vi "Main.vi"() -> ()   [LabVIEW 2015]
doc: "Use this template to build a simple state machine design pattern. Each state executes code and determines which state to transition to."
uses:
  controls/Data.ctl
  <vilib>/MakerHub/LINX/Private/Type Defs/LINX Ref.ctl
  <vilib>/MakerHub/LINX/Private/Type Defs/Platform.ctl
  <vilib>/MakerHub/LINX/Private/Type Defs/Interface.ctl
  <vilib>/MakerHub/LINX/Private/Device/Type Defs/LINX Device Config.ctl
  <vilib>/MakerHub/LINX/Private/Device/Type Defs/TCP Config.ctl
  <vilib>/MakerHub/LINX/Private/Device/Type Defs/Channels.ctl
  controls/State.ctl
  <vilib>/userdefined/High Color/IMAQdx.ctl
  <vilib>/vision/Avi.llb/IMAQ AVI2 Refnum.ctl
  <vilib>/vision/Avi.llb/IMAQ AVI2 Codec Path.ctl
  <vilib>/vision/driver/IMAQdx.llb/IMAQdx Camera Control Mode.ctl
  <vilib>/MakerHub/LINX/Private/Type Defs/User Platform.ctl
  <vilib>/MakerHub/LINX/Public/Peripherals/Digital/Digital Write 1 Chan.vi
  <vilib>/MakerHub/LINX/Public/Peripherals/Digital/Digital Write N Chans.vi
  <vilib>/MakerHub/LINX/Private/Local IO/LinxDigitalWrite.vi
  <vilib>/MakerHub/LINX/Public/Utilities/Check Channel.vi
  <vilib>/Instr/_visa.llb/VISA Configure Serial Port (Instr).vi
  <vilib>/MakerHub/LINX/Private/Utilties/Generate Error.vi
  <vilib>/MakerHub/LINX/LMH-LINX.lvlib
  <vilib>/vision/driver/NI_Vision_Acquisition_Software.lvlib
  <vilib>/measure/NI_MABase.lvlib
  <vilib>/MakerHub/LINX/Private/Device/Device.lvlib
panel:
  in  "Camera":T1="cam1"
  in  "Change Hopper Angle":bool
  in  "Hopper Angle":dbl=90.0
  in  "Left Hole Servo ID":u8=8
  in  "Right Hole Servo ID":u8=11
  in  "Table Tilt Servo ID":u8
  out "Current State":T2
  out "Data":T3={"LED"=FALSE, "Current State "="", "Current Angle"=0.0, "Angle Offset"=0.0, "Motor COM"="COM3", "Table Angle"=0.0, "LINX Ref"={"IO"=enum."Remote", "Interface"=enum."Serial", "LINX Device Config"={"Interface"=enum."Serial", "COM Port"="", "TCP Configuration"={"IP Address"="", "Port"=0}, "Device Family"=0, "Device ID"=0, "Device Name"="", "TCP Ref"=refnum, "Channels"={"DI"=[], "DO"=[], "AI"=[], "AO"=[], "PWM"=[], "QE"=[], "UART"=[], "I2C 2"=[], "SPI"=[], "CAN"=[], "Servo"=[], "AI Ref (V)"=0.0, "AI Resolution (Bits)"=0, "AO Ref (V)"=0.0, "AO Resolution (Bits)"=0}}}, "Mag-Filtered"={"X Axis"=0.0, "Y Axis"=0.0, "Z Axis"=0.0}, "G-Filtered"={"X Axis"=0.0, "Y Axis"=0.0, "Z Axis"=0.0}, "Desired Angle"=0.0, "Run Index"=0}
  in  "Start Automation":bool
  in  "Table Angle Array":dbl[](array[numeric])
  in  "Light LED":bool
  in  "Accelerometer Samples":i32=10
  in  "Save Frames":bool
  in  "Servo Incr":dbl=0.25
  in  "alpha":dbl=0.5 format="%#_13g"
  in  "Chip":enum16{"LSM6DS1", "LSM6DS3", "ADXL345"}(ring)=enum."ADXL345"
  in  "End video":bool=TRUE
  out "Start Video":bool=TRUE
  out "actual path":path
  out "Error Out":errorcluster
  out "Start Camera":bool=TRUE
  out "Camera In":T10(plugin-control)
  in  "Recalibrate":bool
  out "Current Table Angle":dbl
  in  "Motor COM":refnum<visa-resource-name>="COM10"
  in  "Arduino COM":refnum<visa-resource-name>="COM9"
  out "Device Name":string
  in  "Angle":dbl
  out "Current Servo Angle":dbl
  in  "Move To Angle":bool
  out "Exit":bool
  # "-90"
  # "-90"
  # "90"
  # "90"
  # "72 is FLAT!!!"
  # "Sim Controls"
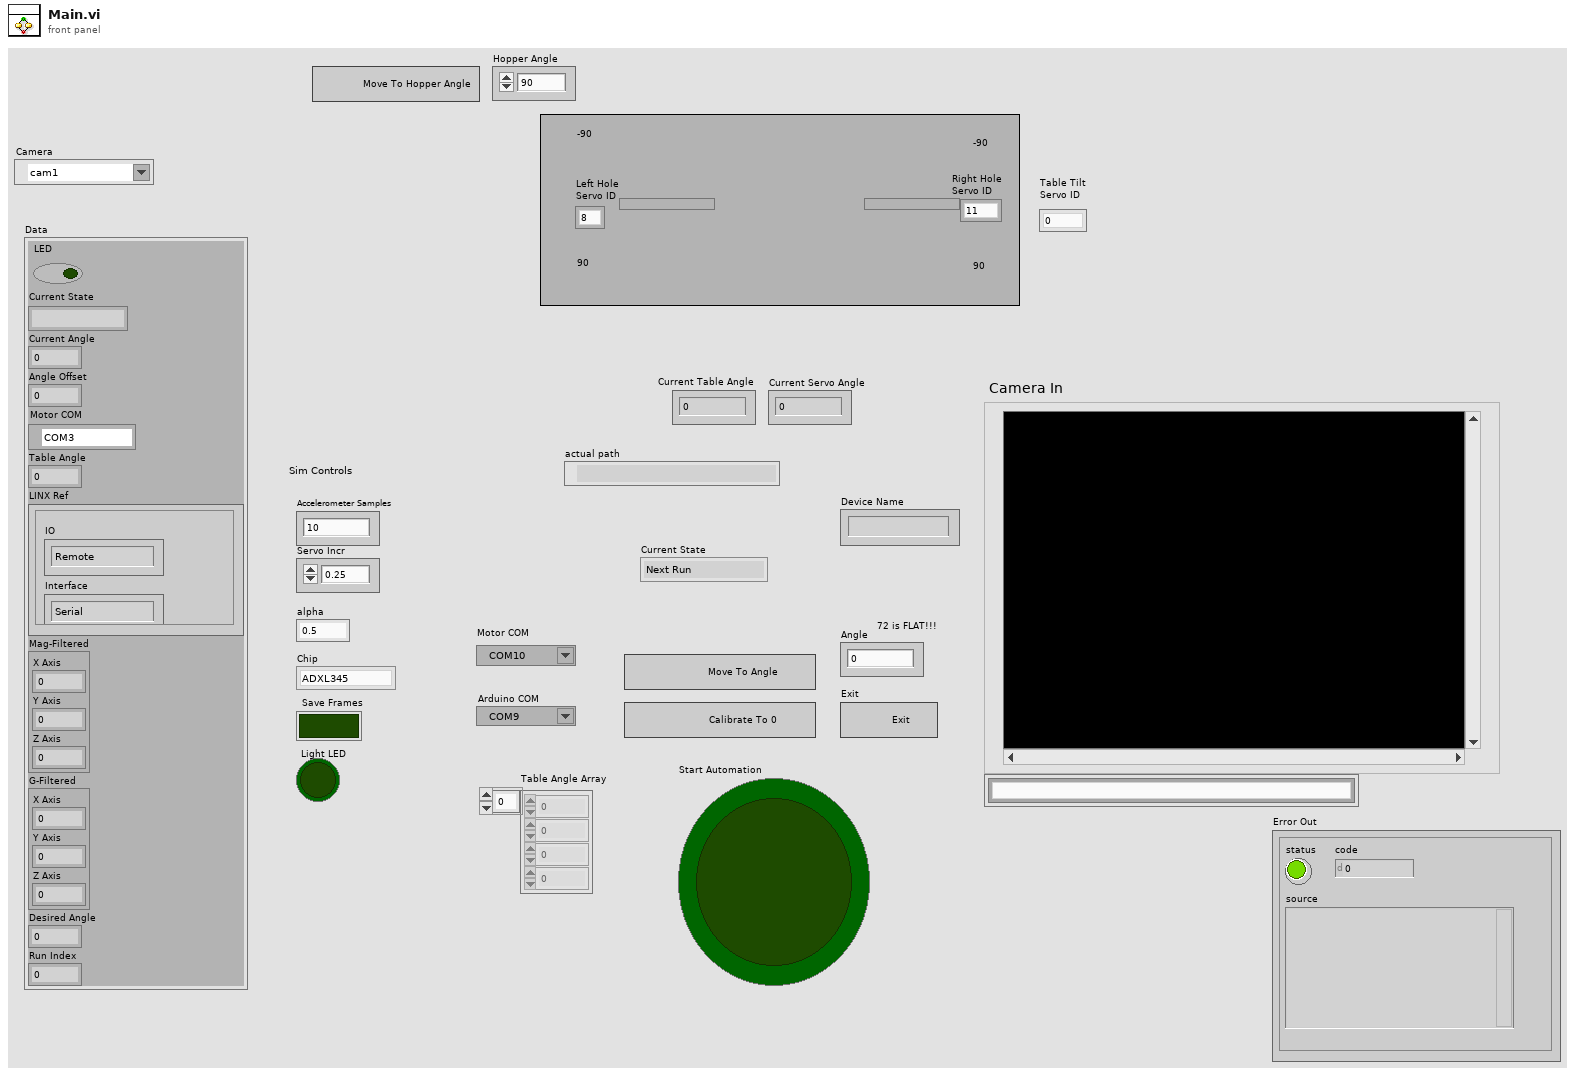
[diagram p1: front panel]
types:
  T1 = typedef "IMAQdx.ctl" = refnum<k21>
  T2 = typedef "State.ctl" = enum16{"Next Run", "Move To Angle (Auto)", "Initialize", "Initialize Camera", "Start Accelerometer", "Wait for Event", "User State 1", "User State 2", "Calibrate Angle", "Change Hole Angle", "Get Accelerometer Angle", "Move To Angle", "Play Tones", "Start Video", "End Video", "Move to 0", "Exit"}
  T3 = typedef "Data.ctl" = cluster{"LED":bool, "Current State ":string, "Current Angle":dbl, "Angle Offset":dbl, "Motor COM":refnum<visa-resource-name>, "Table Angle":dbl, "LINX Ref":T4, "Mag-Filtered":cluster{"X Axis":dbl, "Y Axis":dbl, "Z Axis":dbl}, "G-Filtered":cluster{"X Axis":dbl, "Y Axis":dbl, "Z Axis":dbl}, "Desired Angle":dbl, "Run Index":i32}
  T4 = typedef "LMH-LINX.lvlib/LINX Ref.ctl" = cluster{"IO":T5, "Interface":T6, "LINX Device Config":T7}
  T5 = typedef "LMH-LINX.lvlib/Platform.ctl" = enum16{"Remote", "Local"}
  T6 = typedef "LMH-LINX.lvlib/Interface.ctl" = enum16{"Serial", "TCP"}
  T7 = typedef "LMH-LINX.lvlib/Device.lvlib/LINX Device Config.ctl" = cluster{"Interface":T6, "COM Port":refnum<visa-resource-name>, "TCP Configuration":T8, "Device Family":u8, "Device ID":u8, "Device Name":string, "TCP Ref":refnum<k5>, "Channels":T9}
  T8 = typedef "LMH-LINX.lvlib/Device.lvlib/TCP Config.ctl" = cluster{"IP Address":string, "Port":u16}
  T9 = typedef "LMH-LINX.lvlib/Channels.ctl" = cluster{"DI":u8[], "DO":u8[], "AI":u8[], "AO":u8[], "PWM":u8[], "QE":u8[], "UART":u8[], "I2C 2":u8[], "SPI":u8[], "CAN":u8[], "Servo":u8[], "AI Ref (V)":dbl, "AI Resolution (Bits)":u8, "AO Ref (V)":dbl, "AO Resolution (Bits)":u8}
  T10 = typedef "IMAQ Image.ctl" = refnum<image>
  T11 = cluster{"X Axis":dbl, "Y Axis":dbl, "Z Axis":dbl}
  T12 = typedef "LMH-LINX.lvlib/User Platform.ctl" = enum16{"Default", "Remote", "Local"}
  T13 = typedef "IMAQ AVI2 Refnum.ctl" = refnum<k20>
  T14 = typedef "NI_Vision_Acquisition_Software.lvlib/IMAQdx Camera Control Mode.ctl" = enum32{"Controller", "Listener"}
  T15 = typedef "IMAQ AVI2 Codec Path.ctl" = u32
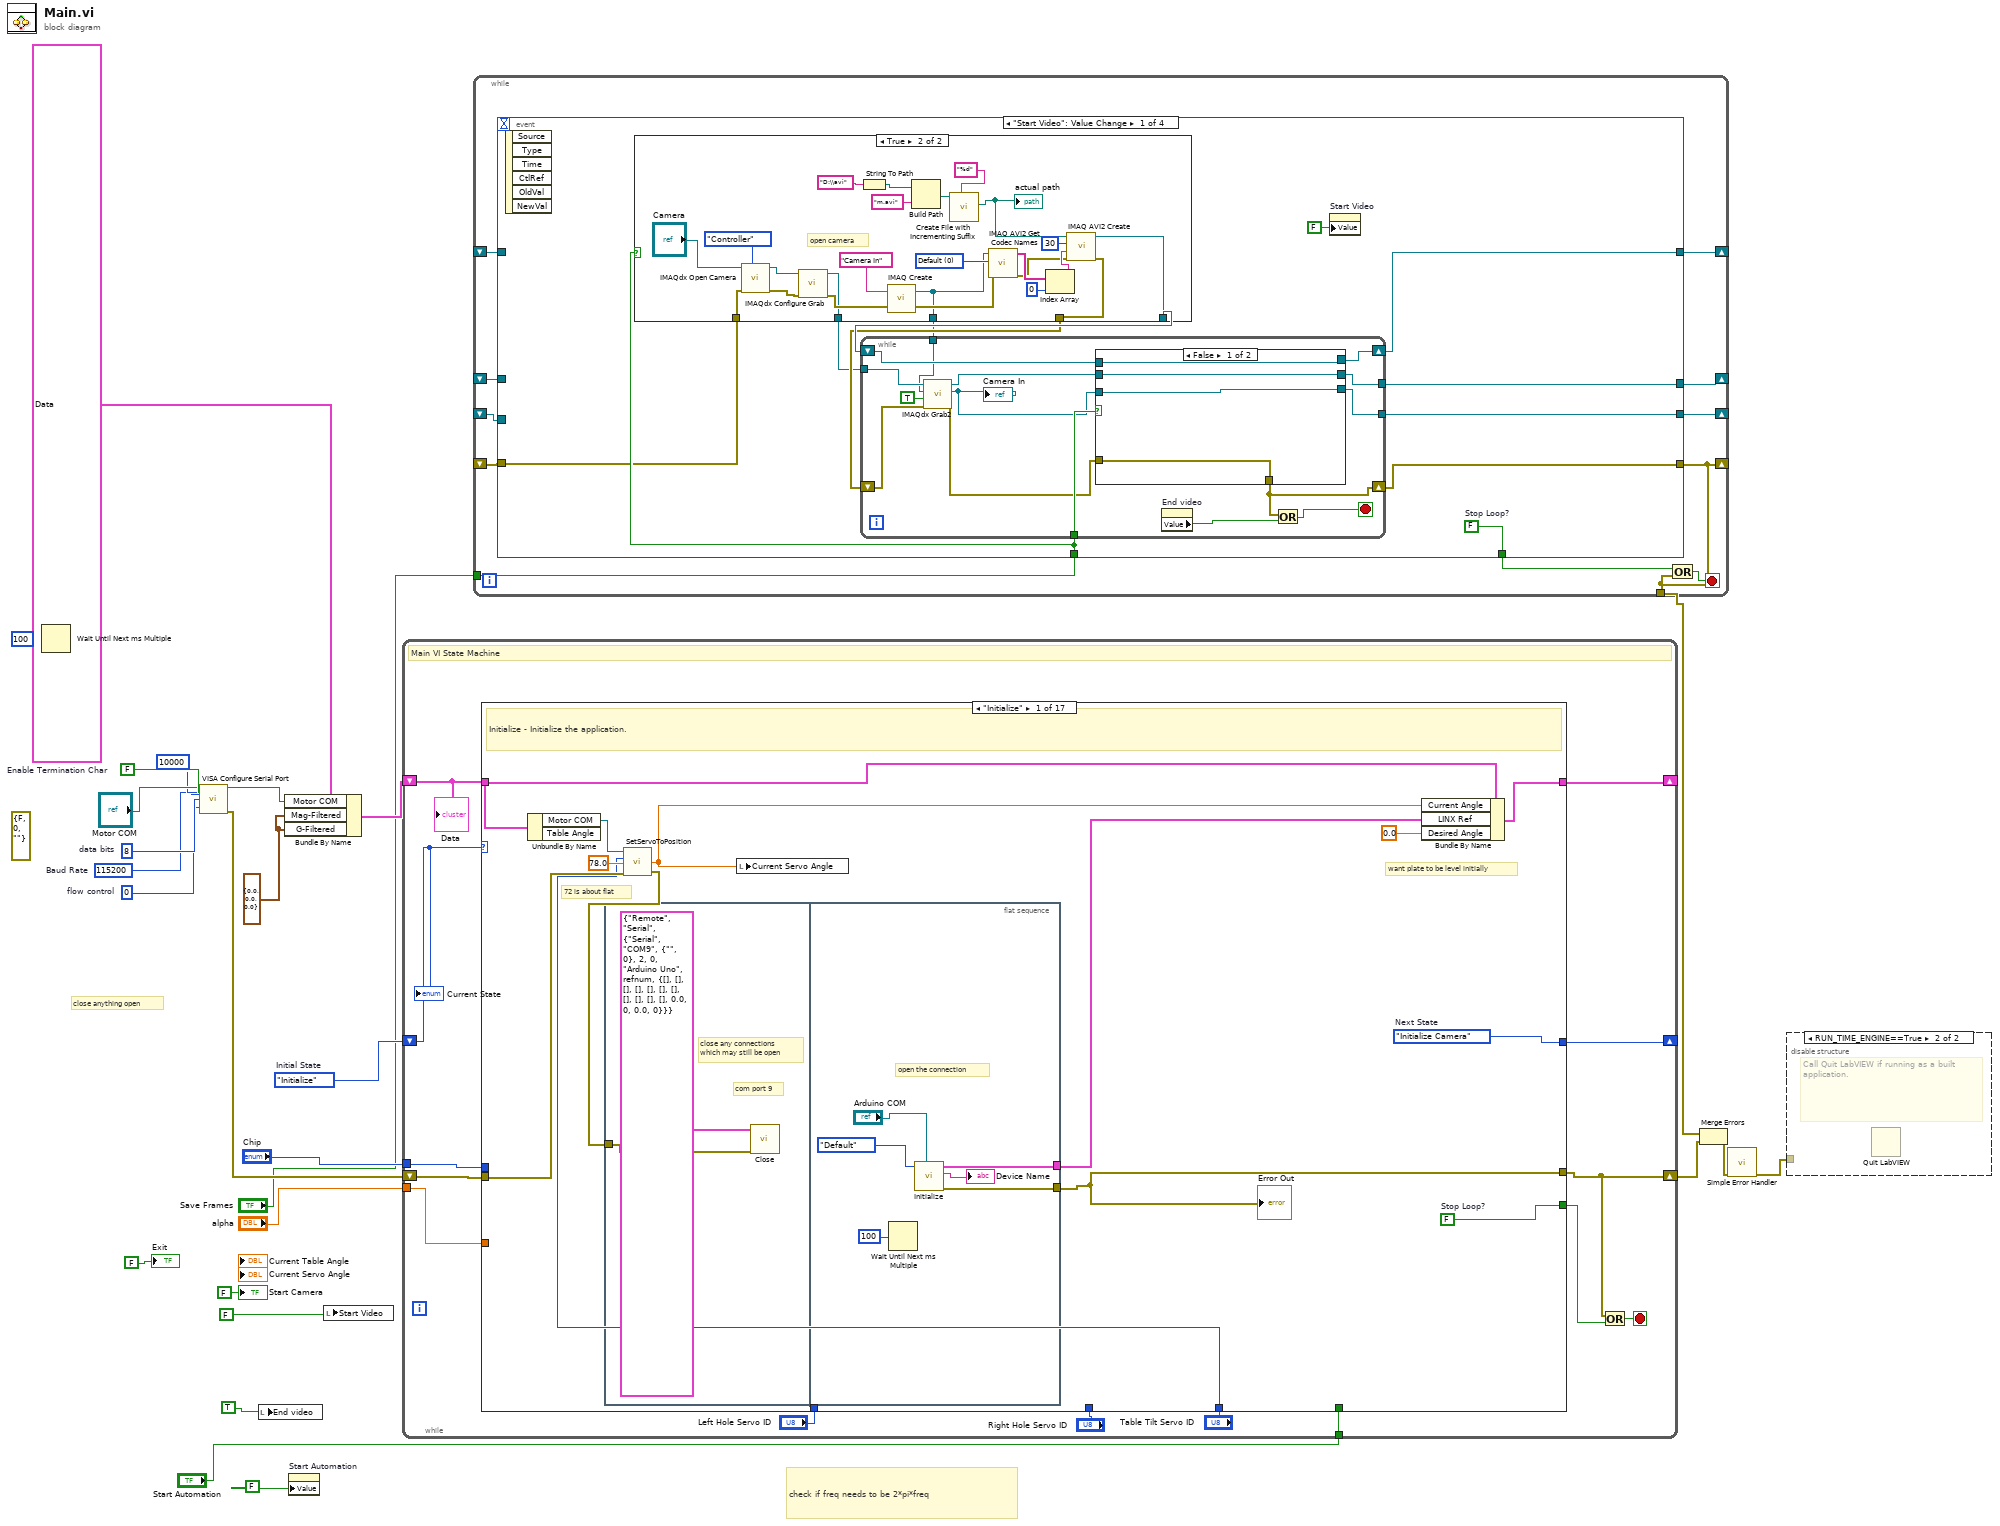
[diagram p0: block diagram]
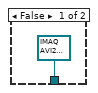
[diagram p2: hidden frame]
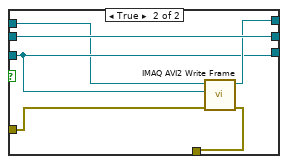
[diagram p3: hidden frame]
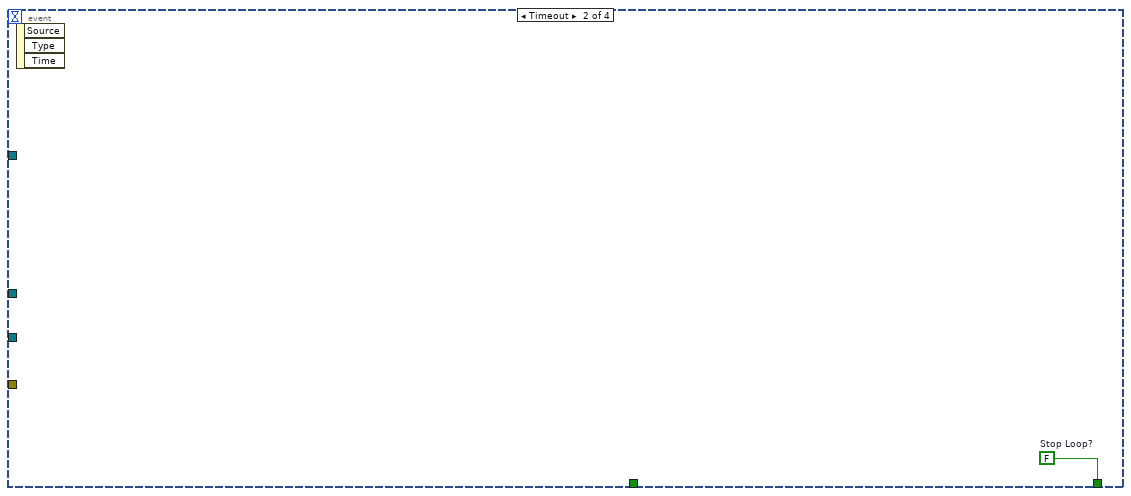
[diagram p4: hidden frame]
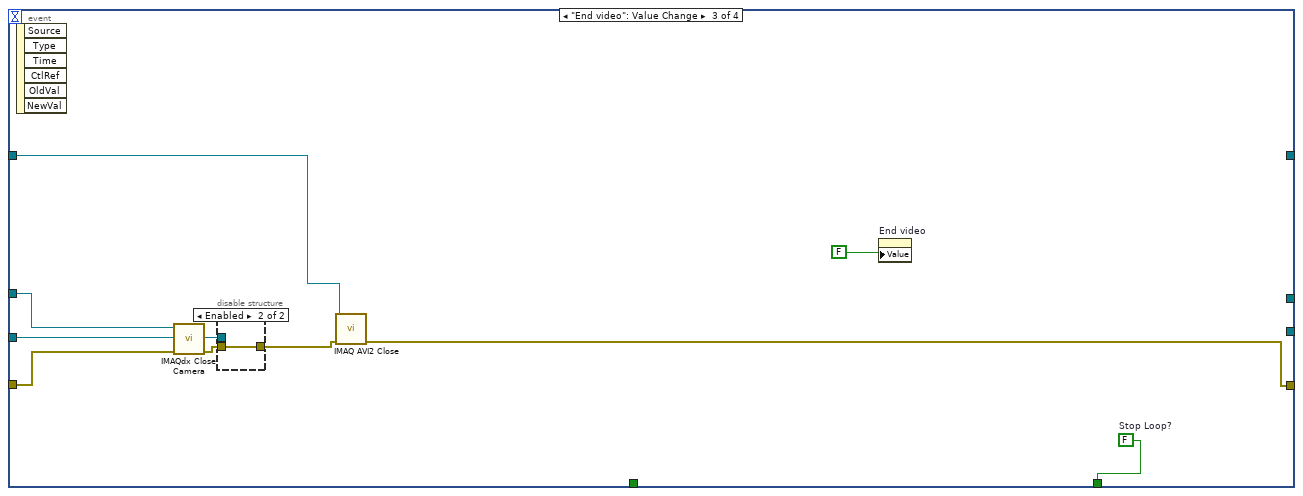
[diagram p5: hidden frame]
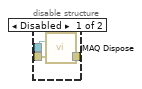
[diagram p6: hidden frame]
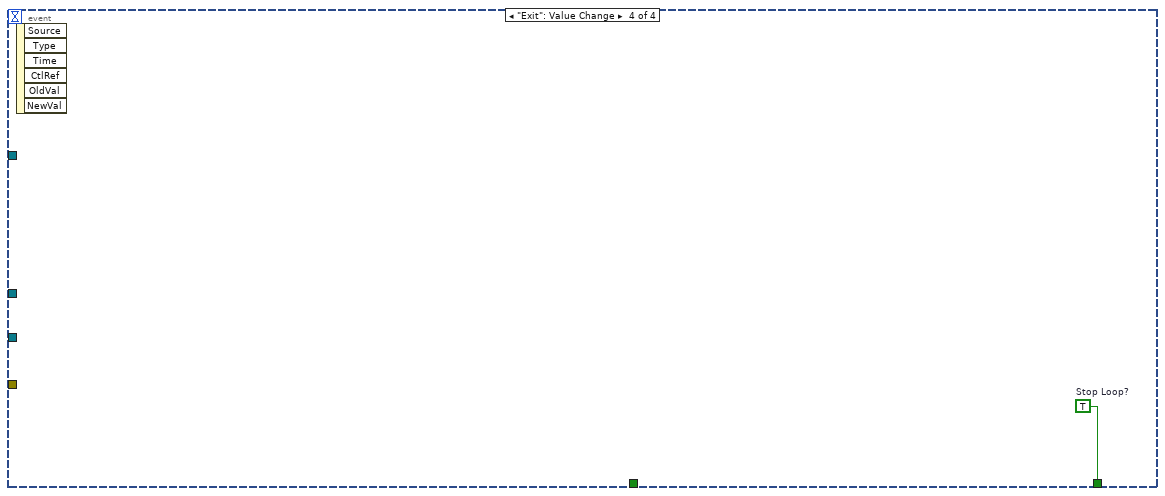
[diagram p7: hidden frame]
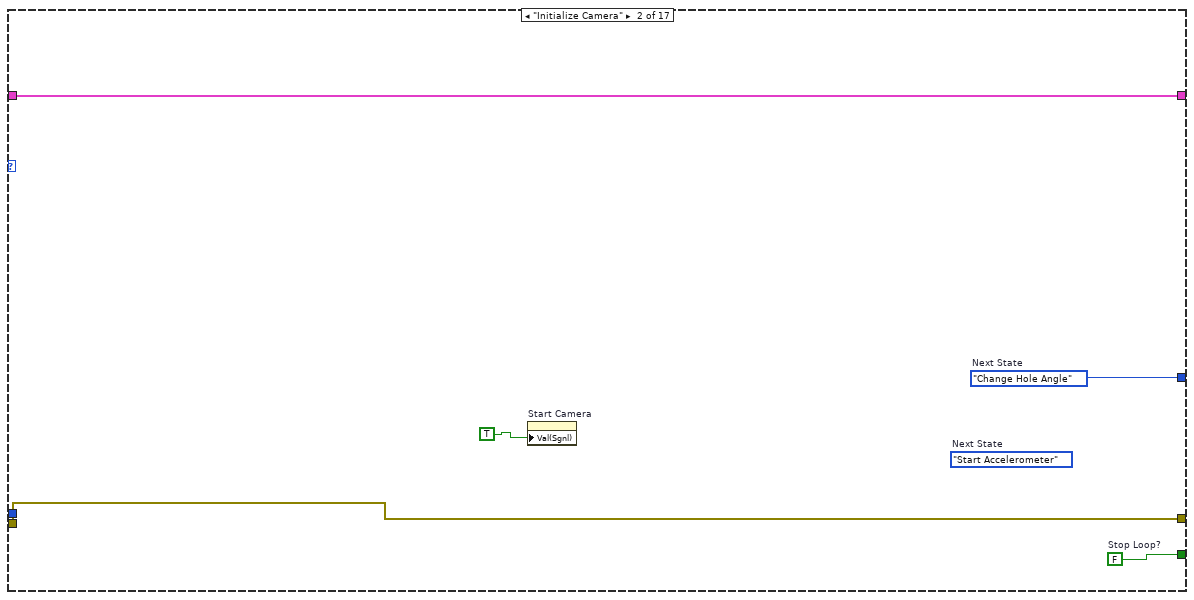
[diagram p9: hidden frame]
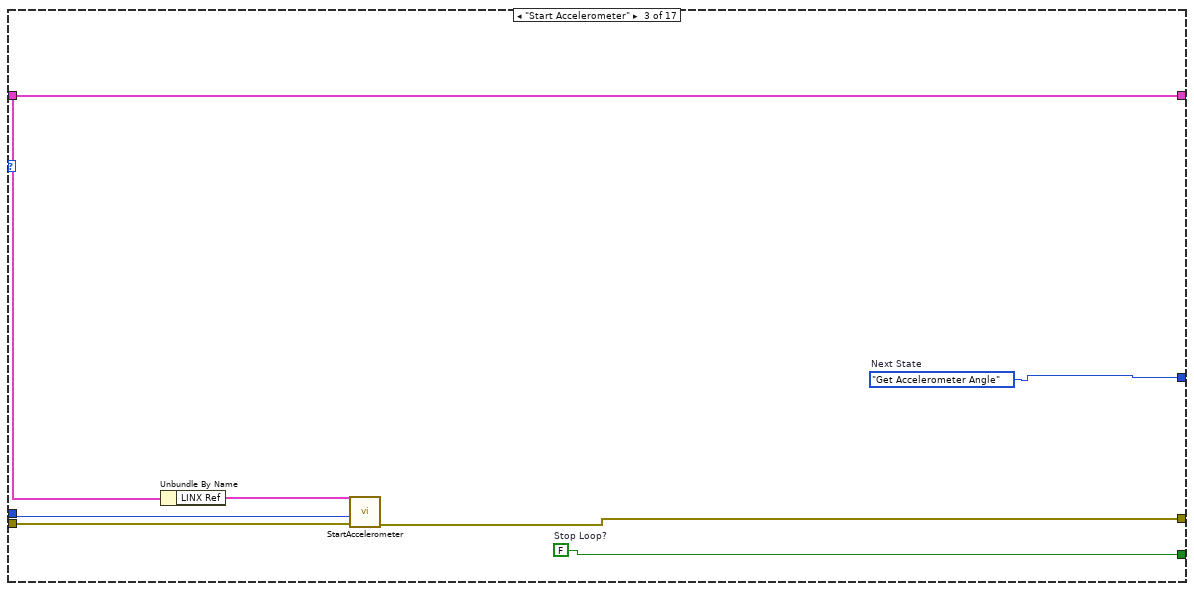
[diagram p10: hidden frame]
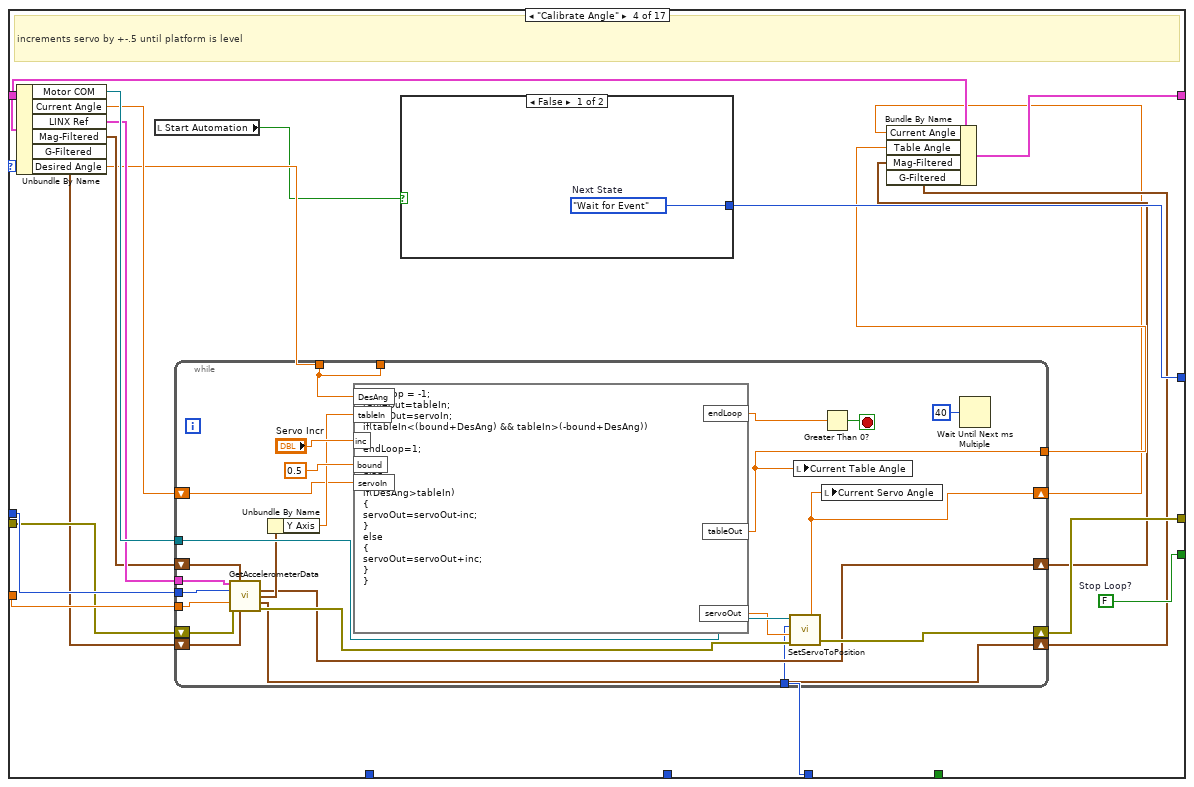
[diagram p11: hidden frame]
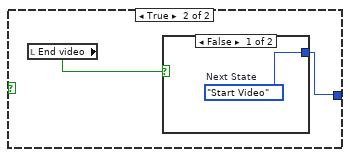
[diagram p12: hidden frame]
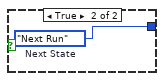
[diagram p13: hidden frame]
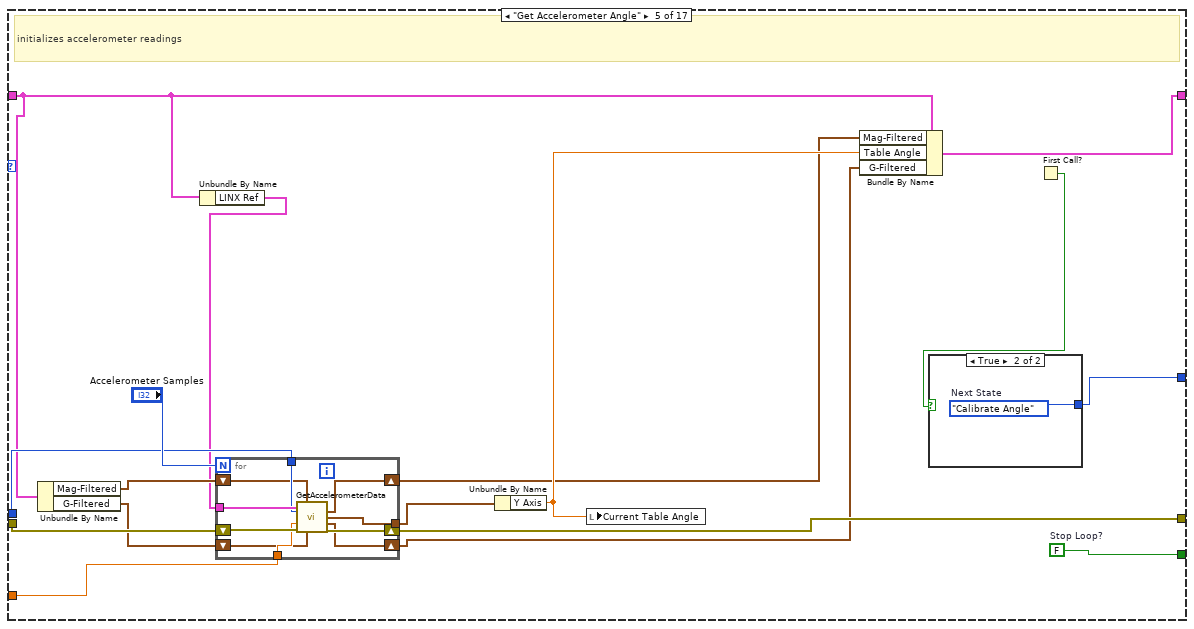
[diagram p14: hidden frame]
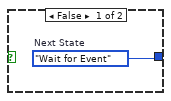
[diagram p15: hidden frame]
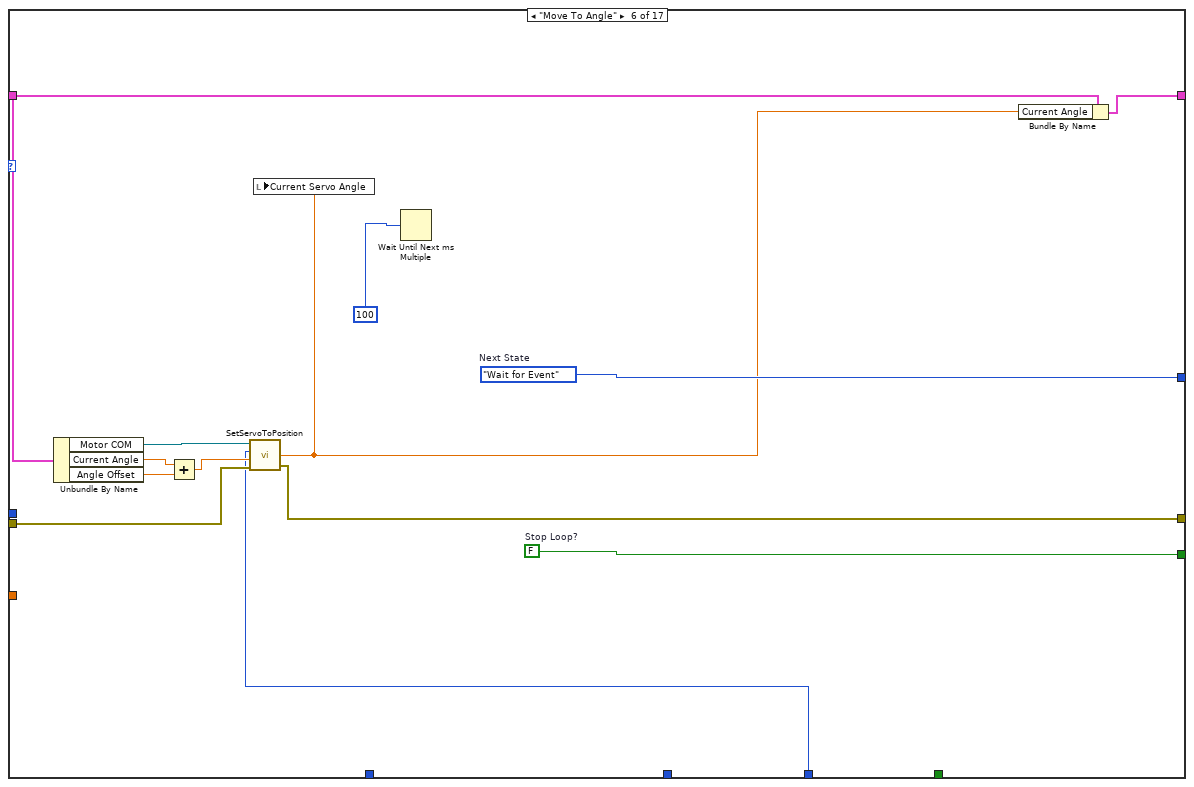
[diagram p16: hidden frame]
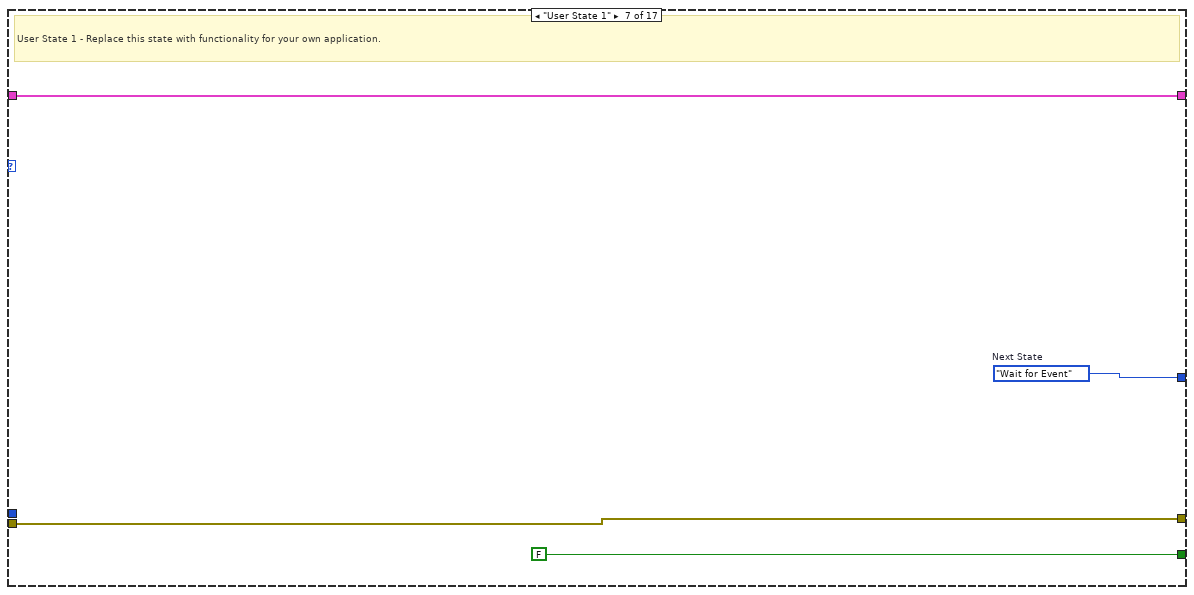
[diagram p17: hidden frame]
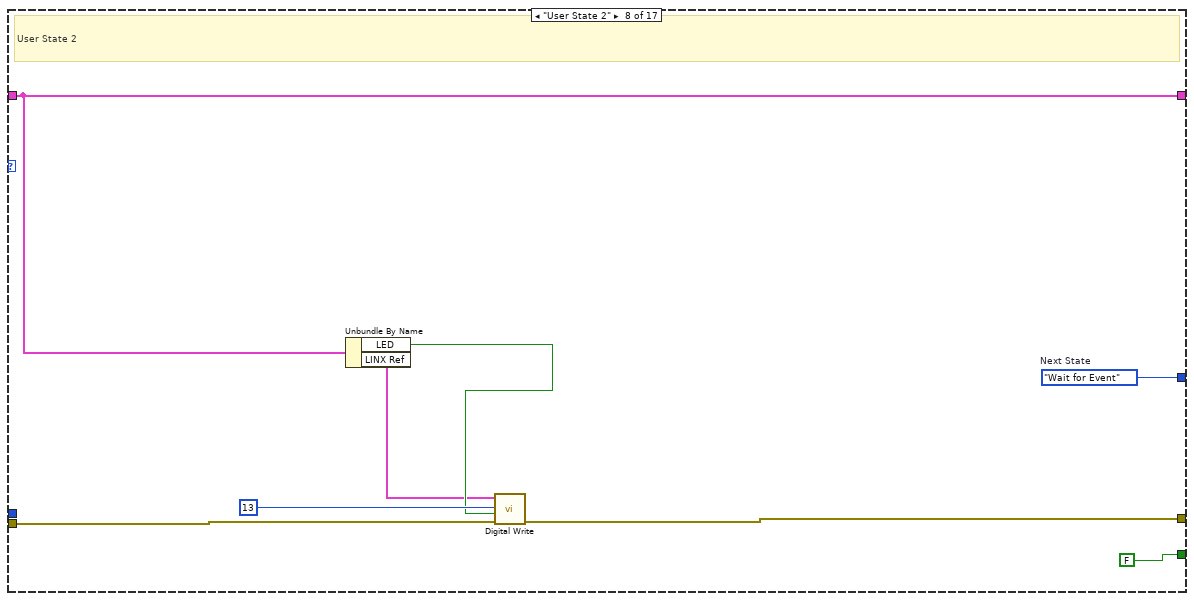
[diagram p18: hidden frame]
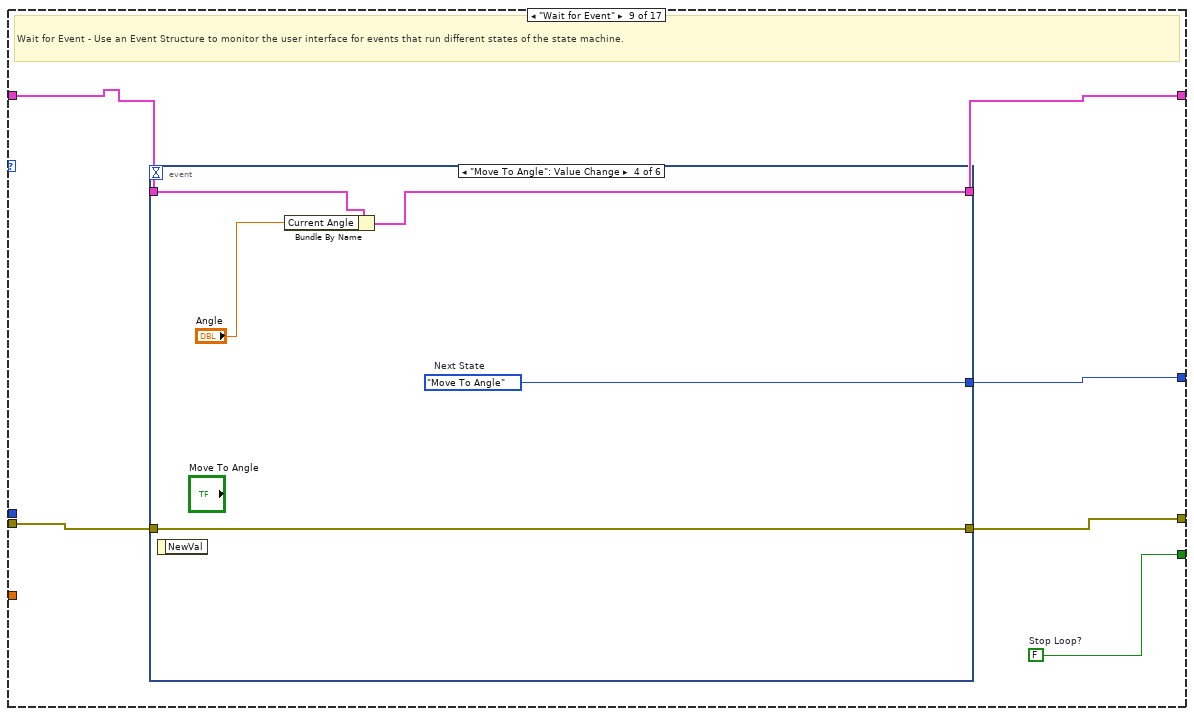
[diagram p19: hidden frame]
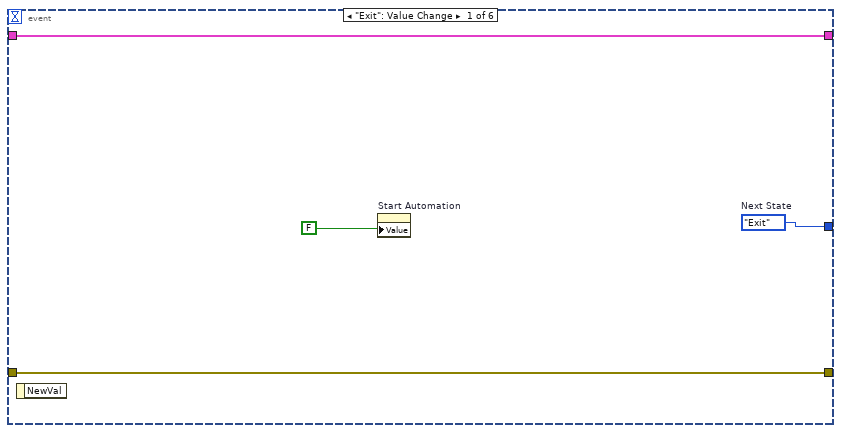
[diagram p20: hidden frame]
diagram:
  w14 = T11 {"X Axis"=0.0, "Y Axis"=0.0, "Z Axis"=0.0} ("Mag-Filtered")
  (unwired) errorcluster {"status"=FALSE, "code"=0, "source"=""} ("error out")
  w8 = u32 115200  # Baud Rate
  w22 = u16 0  # flow control
  w23 = u16 8  # data bits
  w24 = FALSE  # Enable Termination Char
  w20 = State."Initialize"  # Initial State
  # "check if freq needs to be 2*pi*freq"
  # "close anything open"
  n1 = Wait Until Next ms Multiple(millisecond multiple=u32 100) -> ()  [unwired: 1 out]
  n2 = call-poly "VISA Configure Serial Port"("VISA resource name"="Motor COM", "timeout (10sec)"=u32 10000, "Enable Termination\nChar (T)"=w24, "baud rate (9600)"=w8, "data bits (8)"=w23, "flow control (0:none)"=w22) -> ("VISA resource name out"=w7:refnum<visa-resource-name>, "error out"=w21:errorcluster)  [unwired: 8 in]
  n3 = local write "End video"(TRUE ("End video")) -> ()
  n4 = Bundle By Name(cluster=T3 {"LED"=FALSE, "Current State "="", "Current Angle"=0.0, "Angle Offset"=0.0, "Motor COM"="COM3", "Table Angle"=0.0, "LINX Ref"={"IO"=enum."Remote", "Interface"=enum."Serial", "LINX Device Config"={"Interface"=enum."Serial", "COM Port"="", "TCP Configuration"={"IP Address"="", "Port"=0}, "Device Family"=0, "Device ID"=0, "Device Name"="", "TCP Ref"=refnum, "Channels"={"DI"=[], "DO"=[], "AI"=[], "AO"=[], "PWM"=[], "QE"=[], "UART"=[], "I2C 2"=[], "SPI"=[], "CAN"=[], "Servo"=[], "AI Ref (V)"=0.0, "AI Resolution (Bits)"=0, "AO Ref (V)"=0.0, "AO Resolution (Bits)"=0}}}, "Mag-Filtered"={"X Axis"=0.0, "Y Axis"=0.0, "Z Axis"=0.0}, "G-Filtered"={"X Axis"=0.0, "Y Axis"=0.0, "Z Axis"=0.0}, "Desired Angle"=0.0, "Run Index"=0} ("Data"), "Motor COM"=w7, "Mag-Filtered"=w14, "G-Filtered"=w14) -> (w19:T3)
  n5 = property on="Start Automation" class="Bool (strict)"("Value"=FALSE ("End video")) -> ()  [unwired: 2 in, 2 out]
  n6 = local write "Start Video"(FALSE ("Start Video")) -> ()
  n7 = while {
    shift-right: [w40] -> _
    shift-left: w20 -> [w31]
    shift-right: [w39] -> _
    shift-left: w19 -> [w32]
    shift-right: [w35] -> w13
    shift-left: w21 -> [w38]
    tunnel: "Chip" -> [w34]
    tunnel: "alpha" -> [w33]
    tunnel: "Start Automation" -> [w27]
    stop <- w36 stop-if-true
    # "Main VI State Machine"
    n8 = case shown="\"Initialize\"" w31 {
      tunnel: [w53 w65 w67 w91 w138 w163 w168 w176 w182 w211 w224 State."End Video" ("Next State") w249 w264 w291 State."Next Run" ("(Value Not Used)") w308] -> w40
      tunnel: [w52 w66 w73 w93 w139 w164 FALSE ("Stop Loop?") FALSE ("Stop Loop?") w181 w222 w223 w235 w248 w265 w290 _ _] -> w37
      tunnel: w32 -> [w48 w64 w71 w87 w124 w158 w165 w169 w177 w213 w226 w237 w251 w259 w286 w293 w312]
      tunnel: [w49 w64 w71 w92 w130 w162 w165 w169 w180 w217 w226 w237 w251 w255 w286 w292 w312] -> w39
      tunnel: w38 -> [w46 w63 w69 w88 w136 w160 w166 w174 w179 w216 w225 w231 w250 w266 w288 w297 w318]
      tunnel: [w41 w63 w68 w85 w135 w159 w166 w173 w178 w215 w225 w230 w250 w266 w289 w297 w310] -> w35
      tunnel: w34 -> [_ _ w72 w90 w134 _ _ _ _ _ _ _ _ _ _ _ _]
      tunnel: w33 -> [_ _ _ w89 w133 _ _ _ _ _ _ _ _ _ _ _ _]
      tunnel: "Table Tilt Servo ID" -> [w42 _ _ w74 _ w152 _ _ _ w210 _ _ _ _ _ _ _]
      tunnel: "Right Hole Servo ID" -> [_ _ _ _ _ _ _ _ _ _ _ _ _ _ _ _ w319]
      tunnel: "Left Hole Servo ID" -> [_ _ _ _ _ _ _ _ _ _ _ _ _ _ _ _ w315]
      tunnel: w27 -> [_ _ _ _ _ _ _ _ _ _ _ w229 _ _ _ _ _]
      frame "Initialize" {
        w52 = FALSE  # Stop Loop?
        w53 = State."Initialize Camera"  # Next State
        # "want plate to be level initially"
        # "72 is about flat"
        # "Initialize - Initialize the application."
        n9 = Unbundle By Name(w48) -> ("Motor COM"=w50:refnum<visa-resource-name>)  [unwired: 1 out]
        n10 = flat-sequence {
          tunnel: w45 -> [w54]
          tunnel: [w58] -> w41
          tunnel: [w57] -> w44
          frame #0 {
            # "com port 9"
            # "close any connections\nwhich may still be open"
            n11 = call <vilib>:"Close.vi"("Error In"=w54, "LINX Resource"=T4 {"IO"=enum."Remote", "Interface"=enum."Serial", "LINX Device Config"={"Interface"=enum."Serial", "COM Port"="COM9", "TCP Configuration"={"IP Address"="", "Port"=0}, "Device Family"=2, "Device ID"=0, "Device Name"="Arduino Uno", "TCP Ref"=refnum, "Channels"={"DI"=[], "DO"=[], "AI"=[], "AO"=[], "PWM"=[], "QE"=[], "UART"=[], "I2C 2"=[], "SPI"=[], "CAN"=[], "Servo"=[], "AI Ref (V)"=0.0, "AI Resolution (Bits)"=0, "AO Ref (V)"=0.0, "AO Resolution (Bits)"=0}}} ("LINX Ref")) -> ()  [unwired: 9 in, 1 out]
          }
          frame #1 {
            # "open the connection"
            n12 = Wait Until Next ms Multiple(millisecond multiple=u32 100) -> ()  [unwired: 1 out]
            n13 = call <vilib>:"Initialize.vi"("Serial Port"="Arduino COM", "IO"=User_Platform."Default" ("Platform")) -> ("Error Out"=w58:errorcluster, "Device Name"=→"Device Name":string, "LINX Resource"=w57:T4)  [unwired: 7 in]
          }
        }
        n14 = call "SetServoToPosition.vi"("error in (no error)"=w46, "RF LF"=78.0, "servo channel"=w42, "VISA resource name"=w50) -> ("error out"=w45:errorcluster, "RF LF 2"=w47:dbl)  [unwired: 1 out]
        n15 = local write "Current Servo Angle"(w47) -> ()
        n16 = Bundle By Name(cluster=w48, "Current Angle"=w47, "LINX Ref"=w44, "Desired Angle"=0.0) -> (w49:T3)
        "Error Out" <- w41
      }
      frame "Initialize Camera" {
        (unwired) State."Start Accelerometer"  # Next State
        w65 = State."Change Hole Angle"  # Next State
        w66 = FALSE  # Stop Loop?
        n17 = property on="Start Camera" class="Bool (strict)"("Val(Sgnl)"=TRUE) -> ()  [unwired: 2 in, 2 out]
      }
      frame "Start Accelerometer" {
        w67 = State."Get Accelerometer Angle"  # Next State
        w73 = FALSE  # Stop Loop?
        n18 = Unbundle By Name(w71) -> ("LINX Ref"=w70:T4)
        n19 = call "StartAccelerometer.vi"("Error In"=w69, "Chip"=w72, "LINX Resource"=w70) -> ("Error Out"=w68:errorcluster)  [unwired: 3 in, 1 out]
      }
      frame "Calibrate Angle" {
        w93 = FALSE  # Stop Loop?
        # "increments servo by +-.5 until platform is level"
        n20 = Unbundle By Name(w87) -> ("Motor COM"=w86:refnum<visa-resource-name>, "Current Angle"=w84:dbl, "LINX Ref"=w83:T4, "Mag-Filtered"=w81:T11, "G-Filtered"=w79:T11, "Desired Angle"=w77:dbl)
        n21 = local read "Start Automation"() -> (w76:bool)
        n22 = while {
          shift-right: [w101] -> w80
          shift-left: w79 -> [w120]
          tunnel: w90 -> [w119]
          tunnel: w89 -> [w118]
          shift-right: [w109] -> w85
          shift-left: w88 -> [w117]
          shift-right: [w102] -> w78
          shift-left: w81 -> [w115]
          tunnel: w86 -> [w116]
          tunnel: [w106] -> w82
          shift-right: [w104] -> w75
          shift-left: w84 -> [w107]
          tunnel: [w100] -> _
          tunnel: w83 -> [w121]
          tunnel: w77 -> [w100]
          tunnel: w74 -> [w99]
          stop <- w114 stop-if-true
          n23 = call "GetAccelerometerData.vi"("LINX Resource"=w121, "input Mag"=w115, "Chip"=w119, "alpha"=w118, "Error In"=w117, "input Gs"=w120) -> ("Mag-Filtered"=w102:T11, "Roll Pitch Yaw"=w103:T11, "G-Filtered"=w101:T11, "Error Out"=w110:errorcluster)  [unwired: 5 in, 1 out]
          n24 = Unbundle By Name(w103) -> ("Y Axis"=w108:dbl)
          n25 = formula code="endLoop = -1;\ntableOut=tableIn;\nservoOut=servoIn;\nif(tableIn<(bound+DesAng) && tableIn>(-bound+DesAng))\n{\nendLoop=1;\n}\nelse\n{\nif(DesAng>tableIn)\n{\nservoOut=servoOut-inc;\n}\nelse\n{\nservoOut=servoOut+inc;\n}\n}"("tableIn"=w108, "inc"="Servo Incr", "bound"=0.5 ("upper limit"), "servoIn"=w107, "DesAng"=w100) -> ("endLoop"=w111:dbl, "tableOut"=w106:dbl, "servoOut"=w105:dbl)
          n26 = call "SetServoToPosition.vi"("error in (no error)"=w110, "RF LF"=w105, "servo channel"=w99, "VISA resource name"=w116) -> ("error out"=w109:errorcluster, "RF LF 2"=w104:dbl)  [unwired: 1 out]
          n27 = local write "Current Table Angle"(w106) -> ()
          n28 = Greater Than 0?(x=w111) -> (x > 0?=w114:bool)
          n29 = local write "Current Servo Angle"(w104) -> ()
          n30 = Wait Until Next ms Multiple(millisecond multiple=u32 40) -> ()  [unwired: 1 out]
        }
        n31 = case shown="False" w76 {
          tunnel: [w94 w96] -> w91
          frame False {
            w94 = State."Wait for Event"  # Next State
          }
          frame True {
            n32 = local read "End video"() -> (w95:bool)
            n33 = case shown="False" w95 {
              tunnel: [w97 w98] -> w96
              frame False {
                w97 = State."Start Video"  # Next State
              }
              frame True {
                w98 = State."Next Run"  # Next State
              }
            }
          }
        }
        n34 = Bundle By Name(cluster=w87, "Current Angle"=w75, "Table Angle"=w82, "Mag-Filtered"=w78, "G-Filtered"=w80) -> (w92:T3)
      }
      frame "Get Accelerometer Angle" {
        w139 = FALSE  # Stop Loop?
        # "initializes accelerometer readings"
        n35 = Unbundle By Name(w124) -> ("Mag-Filtered"=w129:T11, "G-Filtered"=w128:T11)
        n36 = Unbundle By Name(w124) -> ("LINX Ref"=w123:T4)
        n37 = for {
          N: "Accelerometer Samples" -> [_]
          shift-right: [w149] -> w135
          shift-left: w136 -> [w150]
          tunnel: w134 -> [w148]
          tunnel: w133 -> [w147]
          shift-right: [w143] -> w127
          shift-left: w128 -> [w146]
          shift-right: [w142] -> w125
          shift-left: w129 -> [w145]
          tunnel: [w144] -> w132
          tunnel: w123 -> [w151]
          n38 = call "GetAccelerometerData.vi"("LINX Resource"=w151, "input Mag"=w145, "Chip"=w148, "alpha"=w147, "Error In"=w150, "input Gs"=w146) -> ("Mag-Filtered"=w142:T11, "Roll Pitch Yaw"=w144:T11, "G-Filtered"=w143:T11, "Error Out"=w149:errorcluster)  [unwired: 5 in, 1 out]
        }
        n39 = Unbundle By Name(w132) -> ("Y Axis"=w126:dbl)
        n40 = local write "Current Table Angle"(w126) -> ()
        n41 = Bundle By Name(cluster=w124, "Mag-Filtered"=w125, "Table Angle"=w126, "G-Filtered"=w127) -> (w130:T3)
        n42 = First Call?() -> (First Call?: T/F=w131:bool)
        n43 = case shown="True" w131 {
          tunnel: [w140 w141] -> w138
          frame False {
            w140 = State."Wait for Event"  # Next State
          }
          frame True {
            w141 = State."Calibrate Angle"  # Next State
          }
        }
      }
      frame "Move To Angle" {
        w164 = FALSE  # Stop Loop?
        w163 = State."Wait for Event"  # Next State
        n44 = Unbundle By Name(w158) -> ("Motor COM"=w161:refnum<visa-resource-name>, "Current Angle"=w155:dbl, "Angle Offset"=w154:dbl)
        n45 = Add(x=w155, y=w154) -> (x+y=w153:dbl)
        n46 = call "SetServoToPosition.vi"("error in (no error)"=w160, "RF LF"=w153, "servo channel"=w152, "VISA resource name"=w161) -> ("error out"=w159:errorcluster, "RF LF 2"=w156:dbl)  [unwired: 1 out]
        n47 = local write "Current Servo Angle"(w156) -> ()
        n48 = Wait Until Next ms Multiple(millisecond multiple=u32 100) -> ()  [unwired: 1 out]
        n49 = Bundle By Name(cluster=w158, "Current Angle"=w156) -> (w162:T3)
      }
      frame "User State 1" {
        w168 = State."Wait for Event"  # Next State
        # "User State 1 - Replace this state with functionality for your own application."
      }
      frame "User State 2" {
        w176 = State."Wait for Event"  # Next State
        # "User State 2"
        n50 = Unbundle By Name(w169) -> ("LED"=w171:bool, "LINX Ref"=w170:T4)
        n51 = call-poly <vilib>:"Digital Write.vi"("Error In"=w174, "Output Value"=w171, "DO Channel"=u8 13, "LINX Resource"=w170) -> ("Error Out"=w173:errorcluster)  [unwired: 6 in, 1 out]
      }
      frame "Wait for Event" {
        w181 = FALSE  # Stop Loop?
        # "Wait for Event - Use an Event Structure to monitor the user interface for events that run different states of the state machine."
        n52 = event shown="[3] \"Move To Angle\": Value Change" {
          selector: _ -> [_ _ _ _ _ _]
          dyn-events: _ -> [_ _ _ _ _ _]
          timeout: _ -> [_ _ _ _ _ _]
          tunnel: [w186 w190 w192 w199 w204 w205] -> w182
          tunnel: w177 -> [w185 w189 w194 w197 w202 w207]
          tunnel: [w185 w188 w194 w196 w200 w207] -> w180
          tunnel: w179 -> [w184 w191 w193 w198 w203 w206]
          tunnel: [w184 w191 w193 w198 w203 w206] -> w178
          event "Exit": Value Change {
            w186 = State."Exit"  # Next State
            n53 = event-data() -> ()  [unwired: 1 in, 1 out]
            n54 = property on="Start Automation" class="Bool (strict)"("Value"=FALSE ("End video")) -> ()  [unwired: 2 in, 2 out]
          }
          event "Recalibrate": Value Change {
            w190 = State."Calibrate Angle"  # Next State
            n55 = event-data() -> ()  [unwired: 1 in, 1 out]
            n56 = Bundle By Name(cluster=w189, "Desired Angle"=0.0) -> (w188:T3)
          }
          event "Change Hopper Angle": Value Change {
            w192 = State."Change Hole Angle"  # Next State
            n57 = event-data() -> ()  [unwired: 1 in, 6 out]
          }
          event "Move To Angle": Value Change {
            w199 = State."Move To Angle"  # Next State
            n58 = event-data() -> ()  [unwired: 1 in, 1 out]
            n59 = Bundle By Name(cluster=w197, "Current Angle"="Angle") -> (w196:T3)
          }
          event "Light LED": Value Change {
            w204 = State."User State 2"  # Next State
            n60 = event-data() -> ()  [unwired: 1 in, 1 out]
            n61 = Bundle By Name(cluster=w202, "LED"="Light LED") -> (w200:T3)
          }
          event "Start Automation": Value Change {
            w205 = State."Next Run"  # Next State
            n62 = event-data() -> ()  [unwired: 1 in, 6 out]
          }
        }
      }
      frame "Move To Angle (Auto)" {
        w211 = State."Start Video"  # Initial State
        w222 = FALSE  # Stop Loop?
        n63 = Unbundle By Name(w213) -> ("Motor COM"=w214:refnum<visa-resource-name>, "Run Index"=w208:i32, "Angle Offset"=w219:dbl)
        n64 = Index Array(array="Table Angle Array", index=w208) -> (element=w209:dbl)
        n65 = Add(x=w209, y=w219) -> (x+y=w218:dbl)
        n66 = Wait Until Next ms Multiple(millisecond multiple=u32 100) -> ()  [unwired: 1 out]
        n67 = call "SetServoToPosition.vi"("error in (no error)"=w216, "RF LF"=w218, "servo channel"=w210, "VISA resource name"=w214) -> ("error out"=w215:errorcluster, "RF LF 2"=w220:dbl)  [unwired: 1 out]
        n68 = local write "Current Servo Angle"(w220) -> ()
        n69 = Bundle By Name(cluster=w213, "Current Angle"=w220) -> (w217:T3)
      }
      frame "Start Video" {
        w223 = FALSE  # Stop Loop?
        w224 = State."Play Tones"  # Next State
        # "Start taking data"
        n70 = flat-sequence {
          frame #0 {
            w227 = TRUE
            n71 = property on="Start Video" class="Bool (strict)"("Val(Sgnl)"=w227, "Value"=w227) -> ()  [unwired: 2 in, 2 out]
          }
          frame #1 {
            n72 = Wait (ms)(milliseconds to wait=u32 1000 ("millisecond multiple")) -> ()  [unwired: 1 out]
          }
        }
      }
      frame "Play Tones" {
        w233 = dbl[] [450.0, 225.0, 450.0, 225.0]
        w235 = FALSE  # Stop Loop?
        # "freq"
        # "times"
        # "wait until end?"
        n73 = Array Size(array=w233) -> (size(s)=w234:i32)
        n74 = for {
          N: w234 -> [_]
          tunnel: w233 -> [w242] mode=indexing
          tunnel: dbl[] [5.0, 5.0, 5.0, 5.0] -> [w243] mode=indexing
          shift-right: [w238] -> w230
          shift-left: w231 -> [w239]
          w240 = 8192.0  # sampleRate
          # "# of samp\nsamp freq"
          n75 = Multiply(x=w243, y=w240) -> (x*y=w241:dbl)
          n76 = Bundle By Name(cluster=cluster{"Fs":dbl, "#s":dbl} {"Fs"=8192.0, "#s"=1000.0} ("sampling info"), "#s"=w241, "Fs"=w240) -> (w245:cluster{"Fs":dbl, "#s":dbl})
          n77 = call <vilib>:"Sine Waveform.vi"("sampling info"=w245, "amplitude"=1.0, "frequency"=w242) -> ("signal out"=w247:waveform(dbl))  [unwired: 7 in, 1 out]
          n78 = call "Play Waveform"("Data"=w247, "error in"=w239) -> ("error out"=w238:errorcluster)  [unwired: 17 in]
        }
        n79 = case shown="False" w229 {
          frame False {
          }
          frame True {
          }
        }
      }
      frame "End Video" {
        w248 = FALSE  # Stop Loop?
        w249 = State."Move to 0"  # Next State
        n80 = flat-sequence {
          frame #0 {
            w252 = TRUE ("Value (Signaling)")
            n81 = property on="End video" class="Bool (strict)"("Val(Sgnl)"=w252, "Value"=w252) -> ()  [unwired: 2 in, 2 out]
          }
          frame #1 {
            n82 = Wait (ms)(milliseconds to wait=u32 1000 ("millisecond multiple")) -> ()  [unwired: 1 out]
          }
        }
      }
      frame "Next Run" {
        w265 = FALSE  # Stop Loop?
        # "dont add if first run"
        # "if run index is larger than array"
        n83 = Unbundle By Name(w259) -> ("Run Index"=w261:i32)
        n84 = local read "Table Angle Array"() -> (w263:dbl[])
        n85 = First Call?() -> (First Call?: T/F=w257:bool)
        n86 = case shown="True" w257 {
          tunnel: w261 -> [w268 w269]
          tunnel: [w267 w269] -> w258
          frame False {
            n87 = Increment(x=w268) -> (x+1=w267:i32)
          }
          frame True {
          }
        }
        n88 = Array Size(array=w263) -> (size(s)=w262:i32)
        n89 = property on="End video" class="Bool (strict)"("Value"=FALSE ("Value (Signaling)")) -> ()  [unwired: 2 in, 2 out]
        n90 = Greater Or Equal?(x=w258, y=w262) -> (x >= y?=w260:bool)
        n91 = Bundle By Name(cluster=w259, "Run Index"=w258) -> (w256:T3)
        n92 = case shown="False" w260 {
          tunnel: [State."Change Hole Angle" ("Next State") State."Exit" ("Next State")] -> w264
          tunnel: w256 -> [w278 w282]
          tunnel: w258 -> [w274 _]
          tunnel: [w276 w282] -> w255
          frame False {
            # "this flips angles between + and - between runs \nworks like runIdx%2*-1*angleOffset"
            n93 = Quotient & Remainder(x=w274, y=2.0) -> (x-y*floor(x/y)=w273:dbl)  [unwired: 1 out]
            n94 = case shown="1" w273 {
              tunnel: [1.0 ("y") -1.0 ("y")] -> w271
              frame 0, Default {
              }
              frame 1 {
              }
            }
            n95 = local read "Table Angle Array"() -> (w277:dbl[])
            n96 = Index Array(array=w277, index=w274) -> (element=w272:dbl)
            n97 = Multiply(x=w272, y=w271) -> (x*y=w270:dbl)
            n98 = Bundle By Name(cluster=w278, "Desired Angle"=w270) -> (w276:T3)
          }
          frame True {
          }
        }
      }
      frame "Exit" {
        w285 = TRUE  # Stop Loop?
        w290 = TRUE  # Stop Loop?
        w291 = State."Exit"  # (Value Not Used)
        # "Exit - Exit the application."
        n99 = Unbundle By Name(w286) -> ("LINX Ref"=w287:T4)
        n100 = call <vilib>:"Close.vi"("Error In"=w288, "LINX Resource"=w287) -> ("Error Out"=w289:errorcluster)  [unwired: 9 in]
        n101 = property on="Start Automation" class="Bool (strict)"("Value"=FALSE ("End video")) -> ()  [unwired: 2 in, 2 out]
        n102 = property on="Exit" class="Bool"("Val(Sgnl)"=w285) -> ()  [unwired: 2 in, 2 out]
      }
      frame "Move to 0" {
        n103 = Wait (ms)(milliseconds to wait=u32 3000) -> ()  [unwired: 1 out]
        n104 = Bundle By Name(cluster=w293, "Desired Angle"=0.0) -> (w292:T3)
      }
      frame "Change Hole Angle" {
        # "0 deg = 90\n-90 deg = 240\n90 deg = -80"
        # "0 deg = 90\n-90 deg = -65\n90 deg = 255"
        # "if desired angle is postive the  hopper opening must  be positive"
        n105 = Unbundle By Name(w312) -> ("Motor COM"=w311:refnum<visa-resource-name>, "Desired Angle"=w302:dbl)
        n106 = flat-sequence {
          tunnel: w318 -> [w337]
          tunnel: [w336] -> w316
          tunnel: w315 -> [w335]
          tunnel: [w334] -> w313
          tunnel: w311 -> [w333]
          tunnel: [w330] -> w305
          tunnel: [w331] -> w303
          tunnel: w300 -> [w330]
          tunnel: [w342] -> w317
          tunnel: w316 -> [w342]
          tunnel: [w340] -> w314
          tunnel: w313 -> [w340]
          tunnel: [w339] -> w306
          tunnel: w305 -> [w339]
          tunnel: [w338] -> w304
          tunnel: w303 -> [w338]
          tunnel: w319 -> [w349]
          tunnel: w317 -> [w348]
          tunnel: w314 -> [w347]
          tunnel: [w346] -> w310
          tunnel: [w345] -> w307
          tunnel: w306 -> [w345]
          tunnel: w304 -> [w344]
          tunnel: w307 -> [w351]
          frame #0 {
            # "left"
            n107 = expression code="(x-(-90))*(255-(-65))/(90-(-90))+(-65)"(w330) -> (w332:dbl)
            n108 = Negate(x=w330) -> (-x=w331:dbl)
            n109 = call "SetServoToPosition.vi"("error in (no error)"=w337, "RF LF"=w332, "servo channel"=w335, "VISA resource name"=w333) -> ("error out"=w336:errorcluster, "VISA resource name out"=w334:refnum<visa-resource-name>)  [unwired: 1 out]
          }
          frame #1 {
            n110 = Wait (ms)(milliseconds to wait=u32 1000) -> ()  [unwired: 1 out]
          }
          frame #2 {
            # "right is -(left)+90 offset"
            n111 = expression code="(x-(-90))*(240-(-80))/(90-(-90))+(-80)"(w344) -> (w343:dbl)
            n112 = call "SetServoToPosition.vi"("error in (no error)"=w348, "RF LF"=w343, "servo channel"=w349, "VISA resource name"=w347) -> ("error out"=w346:errorcluster)  [unwired: 2 out]
          }
          frame #3 {
            n113 = Negate(x=w351) -> (-x=w350:dbl)
            n114 = Wait (ms)(milliseconds to wait=u32 1000) -> ()  [unwired: 1 out]
            n115 = property on="Hopper Angle" class="DigNum (strict)"("Value"=w350) -> ()  [unwired: 2 in, 2 out]
          }
        }
        n116 = Greater Than 0?(x=w302) -> (x > 0?=w301:bool)
        n117 = Add(x="Hopper Angle", y=6.0) -> ()  [unwired: 1 out]
        n118 = case shown="True" w301 {
          tunnel: "Hopper Angle" -> [w321 w322]
          tunnel: [w320 w323] -> w300
          frame False {
            n119 = Absolute Value(x=w321) -> (abs(x)=w320:dbl)
          }
          frame True {
            n120 = Absolute Value(x=w322) -> (abs(x)=w324:dbl)
            n121 = Negate(x=w324) -> (-x=w323:dbl)
          }
        }
        n122 = First Call?() -> (First Call?: T/F=w309:bool)
        n123 = case shown="False" w309 {
          tunnel: [w326 w329] -> w308
          frame False {
            n124 = local read "Start Automation"() -> (w325:bool)
            n125 = case shown="False" w325 {
              tunnel: [State."Wait for Event" ("(Value Not Used)") State."Calibrate Angle" ("(Value Not Used)")] -> w326
              frame False {
              }
              frame True {
              }
            }
          }
          frame True {
            w329 = State."Start Accelerometer"  # Next State
          }
        }
      }
    }
    n126 = Or(x=w35, y=w37) -> (x .or. y?=w36:bool)
    "Data" <- w32
    "Current State" <- w31
  }
  n127 = while {
    tunnel: [w353] -> w11
    tunnel: "Save Frames" -> [w363]
    shift-right: [w353] -> _
    shift-left: _ -> [w362]
    shift-right: [w361] -> _
    shift-left: _ -> [w360]
    shift-right: [w359] -> _
    shift-left: _ -> [w356]
    shift-right: [w358] -> _
    shift-left: _ -> [w357]
    stop <- w354 stop-if-true
    n128 = event shown="[0] \"Start Video\": Value Change" {
      selector: _ -> [_ _ _ _]
      dyn-events: _ -> [_ _ _ _]
      timeout: _ -> [_ _ _ _]
      tunnel: w363 -> [w371 _ _ _]
      tunnel: [w375 _ _ _] -> w359
      tunnel: [w373 _ w428 _] -> w353
      tunnel: w362 -> [w365 _ w433 _]
      tunnel: [w374 _ _ _] -> w358
      tunnel: w356 -> [_ _ w434 _]
      tunnel: w357 -> [_ _ w432 _]
      tunnel: [w370 _ _ _] -> w361
      tunnel: w360 -> [_ _ w430 _]
      tunnel: [w364 w426 w427 w440] -> w355
      event "Start Video": Value Change {
        w364 = FALSE  # Stop Loop?
        n129 = event-data() -> ()  [unwired: 1 in, 6 out]
        n130 = case shown="True" w371 {
          tunnel: [T13 refnum ("AVI Refnum") w394] -> w369
          tunnel: [_ w386] -> w368
          tunnel: [_ w383] -> w367
          tunnel: [_ w382] -> w366
          tunnel: w365 -> [_ w381]
          frame False {
          }
          frame True {
            w398 = T15 0 items=["Default", "System", "Built in Vision"] ("Codec Source")
            # "open camera"
            n131 = call <vilib>:"IMAQdx Open Camera.vi"("Camera Control Mode"=IMAQdx_Camera_Control_Mode."Controller", "error in"=w381, "Session In"="Camera") -> ("error out"=w391:errorcluster, "Session Out"=w392:T1)  [unwired: 7 in]
            n132 = call <vilib>:"IMAQdx Configure Grab.vi"("error in"=w391, "Session In"=w392) -> ("error out"=w388:errorcluster, "Session Out"=w383:T1)  [unwired: 8 in]
            n133 = String To Path(string="D:\\avi") -> (path=w397:path)
            n134 = call "IMAQ Create"("Image Name"="Camera In", "error in (no error)"=w388) -> ("New Image"=w382:T10, "error out"=w384:errorcluster)  [unwired: 3 in]
            n135 = Build Path(base path=w397, name or relative path="m.avi") -> (appended path=w378:path)
            n136 = call "Create File with Incrementing Suffix.vi"("format string (\" (%d)\")"="%d" ("format string (\" (%d)\")"), "file path"=w378) -> ("actual path"=w380:path)  [unwired: 8 in, 1 out]
            "actual path" <- w380
            n137 = call "IMAQ AVI2 Get Codec Names"("error in (no error)"=w384, "Codec Source"=w398, "Image"=w382) -> ("error out"=w387:errorcluster, "Codec Names"=w400:string[])  [unwired: 7 in]
            n138 = Index Array(array=w400, index=0) -> (element=w399:string)
            n139 = call "IMAQ AVI2 Create"("error in (no error)"=w387, "Codec"=w399, "Frames Per Second"=u32 30, "AVI Path"=w380) -> ("error out"=w386:errorcluster, "AVI Refnum"=w394:T13)  [unwired: 6 in]
          }
        }
        n140 = while {
          shift-right: [w403] -> w373
          shift-left: w368 -> [w414]
          tunnel: w367 -> [w415]
          tunnel: [w411] -> w375
          tunnel: [w409] -> w374
          tunnel: w371 -> [w413]
          shift-right: [w408] -> w370
          shift-left: w369 -> [w406]
          tunnel: w366 -> [w402]
          stop <- w407 stop-if-true
          n141 = call <vilib>:"IMAQdx Grab2.vi"("error in"=w414, "Wait for Next Buffer? (Yes)"=TRUE, "Image In"=w402, "Session In"=w415) -> ("error out"=w404:errorcluster, "Image Out"=w410:T10, "Session Out"=w412:T1)  [unwired: 4 in, 1 out]
          "Camera In" <- w410
          n142 = case shown="False" w413 {
            tunnel: w412 -> [w419 w425]
            tunnel: [w419 w425] -> w411
            tunnel: w410 -> [w418 w423]
            tunnel: [w418 w423] -> w409
            tunnel: [w417 w424] -> w408
            tunnel: w406 -> [w417 w422]
            tunnel: w404 -> [w416 w421]
            tunnel: [w416 w420] -> w403
            frame False {
            }
            frame True {
              n143 = call "IMAQ AVI2 Write Frame"("error in (no error)"=w421, "Image"=w423, "AVI Refnum"=w422) -> ("error out"=w420:errorcluster, "AVI Refnum (duplicate)"=w424:T13)  [unwired: 6 in, 1 out]
            }
          }
          n144 = property on="End video" class="Bool (strict)"() -> ("Value"=w405:bool)  [unwired: 2 in, 2 out]
          n145 = Or(x=w403, y=w405) -> (x .or. y?=w407:bool)
        }
        n146 = property on="Start Video" class="Bool (strict)"("Value"=FALSE ("Start Video")) -> ()  [unwired: 2 in, 2 out]
      }
      event Timeout {
        w426 = FALSE  # Stop Loop?
        n147 = event-data() -> ()  [unwired: 1 in, 3 out]
      }
      event "End video": Value Change {
        w427 = FALSE  # Stop Loop?
        n148 = event-data() -> ()  [unwired: 1 in, 6 out]
        n149 = call <vilib>:"IMAQdx Close Camera.vi"("error in"=w433, "Session In"=w434) -> ("error out"=w435:errorcluster)  [unwired: 9 in]
        n150 = disable-structure shown="Enabled" {
          disable-tunnel: w435 -> [w438 w439]
          disable-tunnel: w432 -> [w437 _]
          disable-tunnel: [w436 w439] -> w429
          frame Disabled {
            n151 = call "IMAQ Dispose"("Image"=w437, "error in (no error)"=w438) -> ("error out"=w436:errorcluster)  [unwired: 4 in]
          }
          frame Enabled {
          }
        }
        n152 = call "IMAQ AVI2 Close"("error in (no error)"=w429, "AVI Refnum"=w430) -> ("error out"=w428:errorcluster)  [unwired: 9 in]
        n153 = property on="End video" class="Bool (strict)"("Value"=FALSE) -> ()  [unwired: 2 in, 2 out]
      }
      event "Exit": Value Change {
        w440 = TRUE  # Stop Loop?
        n154 = event-data() -> ()  [unwired: 1 in, 6 out]
      }
    }
    n155 = Or(x=w355, y=w353) -> (x .or. y?=w354:bool)
  }
  n156 = Merge Errors(w11, w13) -> (w12:errorcluster)
  n157 = call <vilib>:"Simple Error Handler.vi"("error in (no error)"=w12) -> ("error out"=w26:errorcluster)  [unwired: 4 in, 4 out]
  n158 = disable-structure shown="RUN_TIME_ENGINE==True" {
    disable-tunnel: w26 -> [_ _]
    frame condition #0 (active) {
    }
    frame condition #1 {
      # "Call Quit LabVIEW if running as a built application."
      n159 = Quit LabVIEW() -> ()  [unwired: 1 in]
    }
  }
  "Start Camera" <- FALSE ("Start Camera")
  "Exit" <- FALSE ("End video")
